vi "Request Synchronous Timestamp.vi"(6 "Ignore Past Updates? (F)":bool, 7 "Timeout In ms (-1)":i32=-1, 8 "error in (no error)":errorcluster, 9 "Type (Timestamp)":timestamp, 10 "Datum Name":string, 11 "IObserver In":refnum<class "IObserver.lvclass">) -> (0 "error out":errorcluster, 1 "timed out?":bool, 2 "Data (Timestamp)":timestamp, 4 "Publication Time":timestamp)   [LabVIEW 2017, in "IObserver.lvlib" / "IObserver.lvclass"]
doc: "DEPRECATED by Request Synchronous Data.vim"
uses:
  <vilib>/gpm_packages/@cs/mva-core/Source/IObserver/IObserver/IObserver.lvclass
  <vilib>/gpm_packages/@cs/mva-core/Source/IObserver/IObserver/IObserver.lvclass/IObserver.ctl
  <vilib>/gpm_packages/@cs/mva-core/Source/SubscriptionPolicy/OneShotSubscription/OneShotSubscription.lvclass/OneShotSubscription.ctl
  <vilib>/gpm_packages/@cs/transport/Source/Concrete/NotifierTransport/NotifierTransport.lvclass/NotifierTransport.ctl
  <vilib>/gpm_packages/@cs/mva-core/Source/IMediator/SubscriptionRequest/SubscriptionRequest.lvclass/SubscriptionRequest.ctl
  <vilib>/gpm_packages/@cs/mva-core/Source/IMediator/IMediator Messages/Subscribe Msg/Subscribe Msg.lvclass/Subscribe Msg.ctl
  <vilib>/gpm_packages/@cs/actor-framework-messages/Source/RoundTripMessage/RoundTripMessage.lvclass/RoundTripMessage.ctl
  <vilib>/ActorFramework/Message Enqueuer/Message Enqueuer.lvclass/Message Enqueuer.ctl
  <vilib>/gpm_packages/@cs/mva-core/Source/IMediator/SubscriptionRequest/Pack Subscription Request.vi
  <vilib>/gpm_packages/@cs/mva-core/Source/SubscriptionPolicy/OneShotSubscription/New One-Shot Subscription.vi
  <vilib>/gpm_packages/@cs/mva-core/Source/IMediator/IMediator Messages/Subscribe Msg/Send Pre-Addressed Subscribe.vi
  <vilib>/gpm_packages/@cs/transport/Source/Concrete/NotifierTransport/Construct Notifier Transport.vi
  <vilib>/gpm_packages/@cs/transport/Source/Concrete/NotifierTransport/Wait on Transport Notification.vi
  <vilib>/gpm_packages/@cs/actor-framework-messages/Source/RoundTripMessage/Return Round-Trip Message.vi
  <vilib>/ActorFramework/Message Enqueuer/Enqueue.vi
  <vilib>/gpm_packages/@cs/transport/Source/Concrete/NotifierTransport/NotifierTransport.lvclass
  C:/Program Files/National Instruments/LabVIEW 2017/vi.lib/gpm_packages/@cs/transport/Source/ITransport/ITransport.lvclass
  <vilib>/gpm_packages/@cs/mva-core/Source/SubscriptionPolicy/OneShotSubscription/OneShotSubscription.lvclass
  C:/Program Files/National Instruments/LabVIEW 2017/vi.lib/gpm_packages/@cs/mva-core/Source/IMediator/ISubscriptionPolicy/ISubscriptionPolicy.lvclass
  <vilib>/gpm_packages/@cs/mva-core/Source/IMediator/IMediator Messages/Subscribe Msg/Subscribe Msg.lvclass
  C:/Program Files/National Instruments/LabVIEW 2017/vi.lib/gpm_packages/@cs/actor-framework-messages/Source/RoundTripMessage/RoundTripMessage.lvclass
  <vilib>/gpm_packages/@cs/actor-framework-messages/Source/RoundTripMessage/RoundTripMessage.lvclass
  C:/Program Files/National Instruments/LabVIEW 2017/vi.lib/ActorFramework/Message/Message.lvclass
  <vilib>/Utility/error.llb/Error Cluster From Error Code.vi
  <vilib>/ActorFramework/Message Priority Queue/Priority Enqueue.vi
  <vilib>/gpm_packages/@cs/mva-core/Source/IMediator/ISubscriptionPolicy/Open Subscription Policy.vi
  <vilib>/gpm_packages/@cs/mva-core/Source/IMediator/SubscriptionRequest/SubscriptionRequest.lvclass
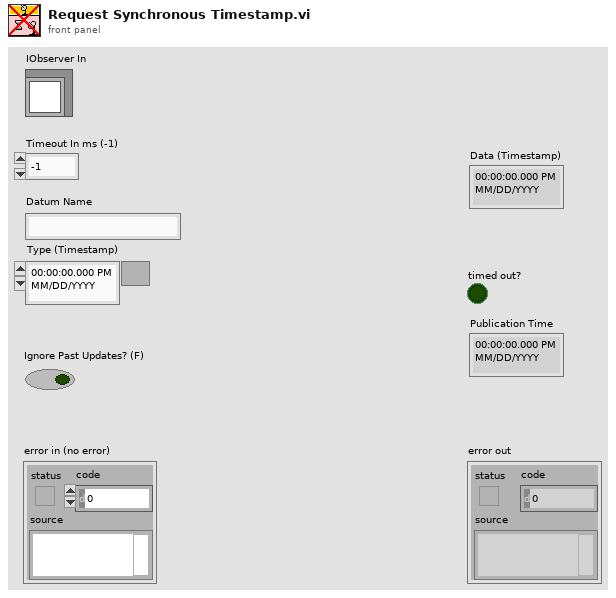
[diagram p1: front panel]
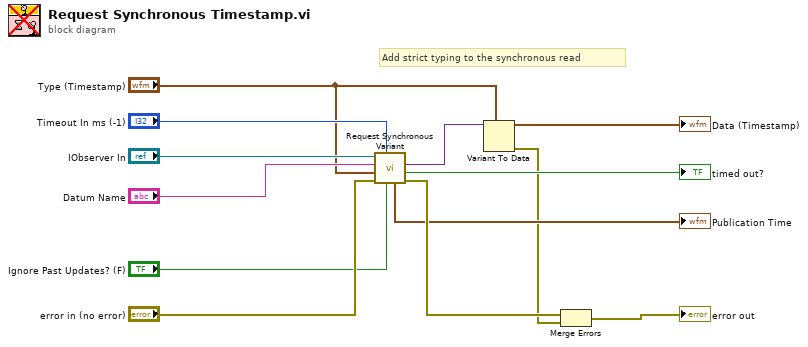
[diagram p0: block diagram]
diagram:
  # "Add strict typing to the synchronous read"
  n1 = call <vilib>:"Request Synchronous Variant.vi"("Ignore Past Updates? (F)"="Ignore Past Updates? (F)", "Timeout In ms (-1)"="Timeout In ms (-1)", "error in (no error)"="error in (no error)", "Type"="Type (Timestamp)", "Datum Name"="Datum Name", "IObserver In"="IObserver In") -> ("error out"=w10:errorcluster, "timed out?"=→"timed out?":bool, "Data"=w6:variant, "Publication Time"=→"Publication Time":timestamp)  [unwired: 2 in]
  n2 = Variant To Data(type="Type (Timestamp)", Variant=w6) -> (data=→"Data (Timestamp)":timestamp, error out=w1:errorcluster)  [unwired: 1 in]
  n3 = Merge Errors(w10, w1) -> (→"error out":errorcluster)
